vi "测试状态判断.vi"(10 "配置信息":T11, 11 "Display State In":T1) -> (1 "Data In":T3 caption="数据", 2 "配置信息读取":T11, 3 "Display State Out":T1)   [LabVIEW 2016, in "定时设置.xctl"]
uses:
  <vilib>/ptbypt/NI_PtbyPt.lvlib
panel:
  # "分钟"
  # "次"
  # "分钟"
  # "次"
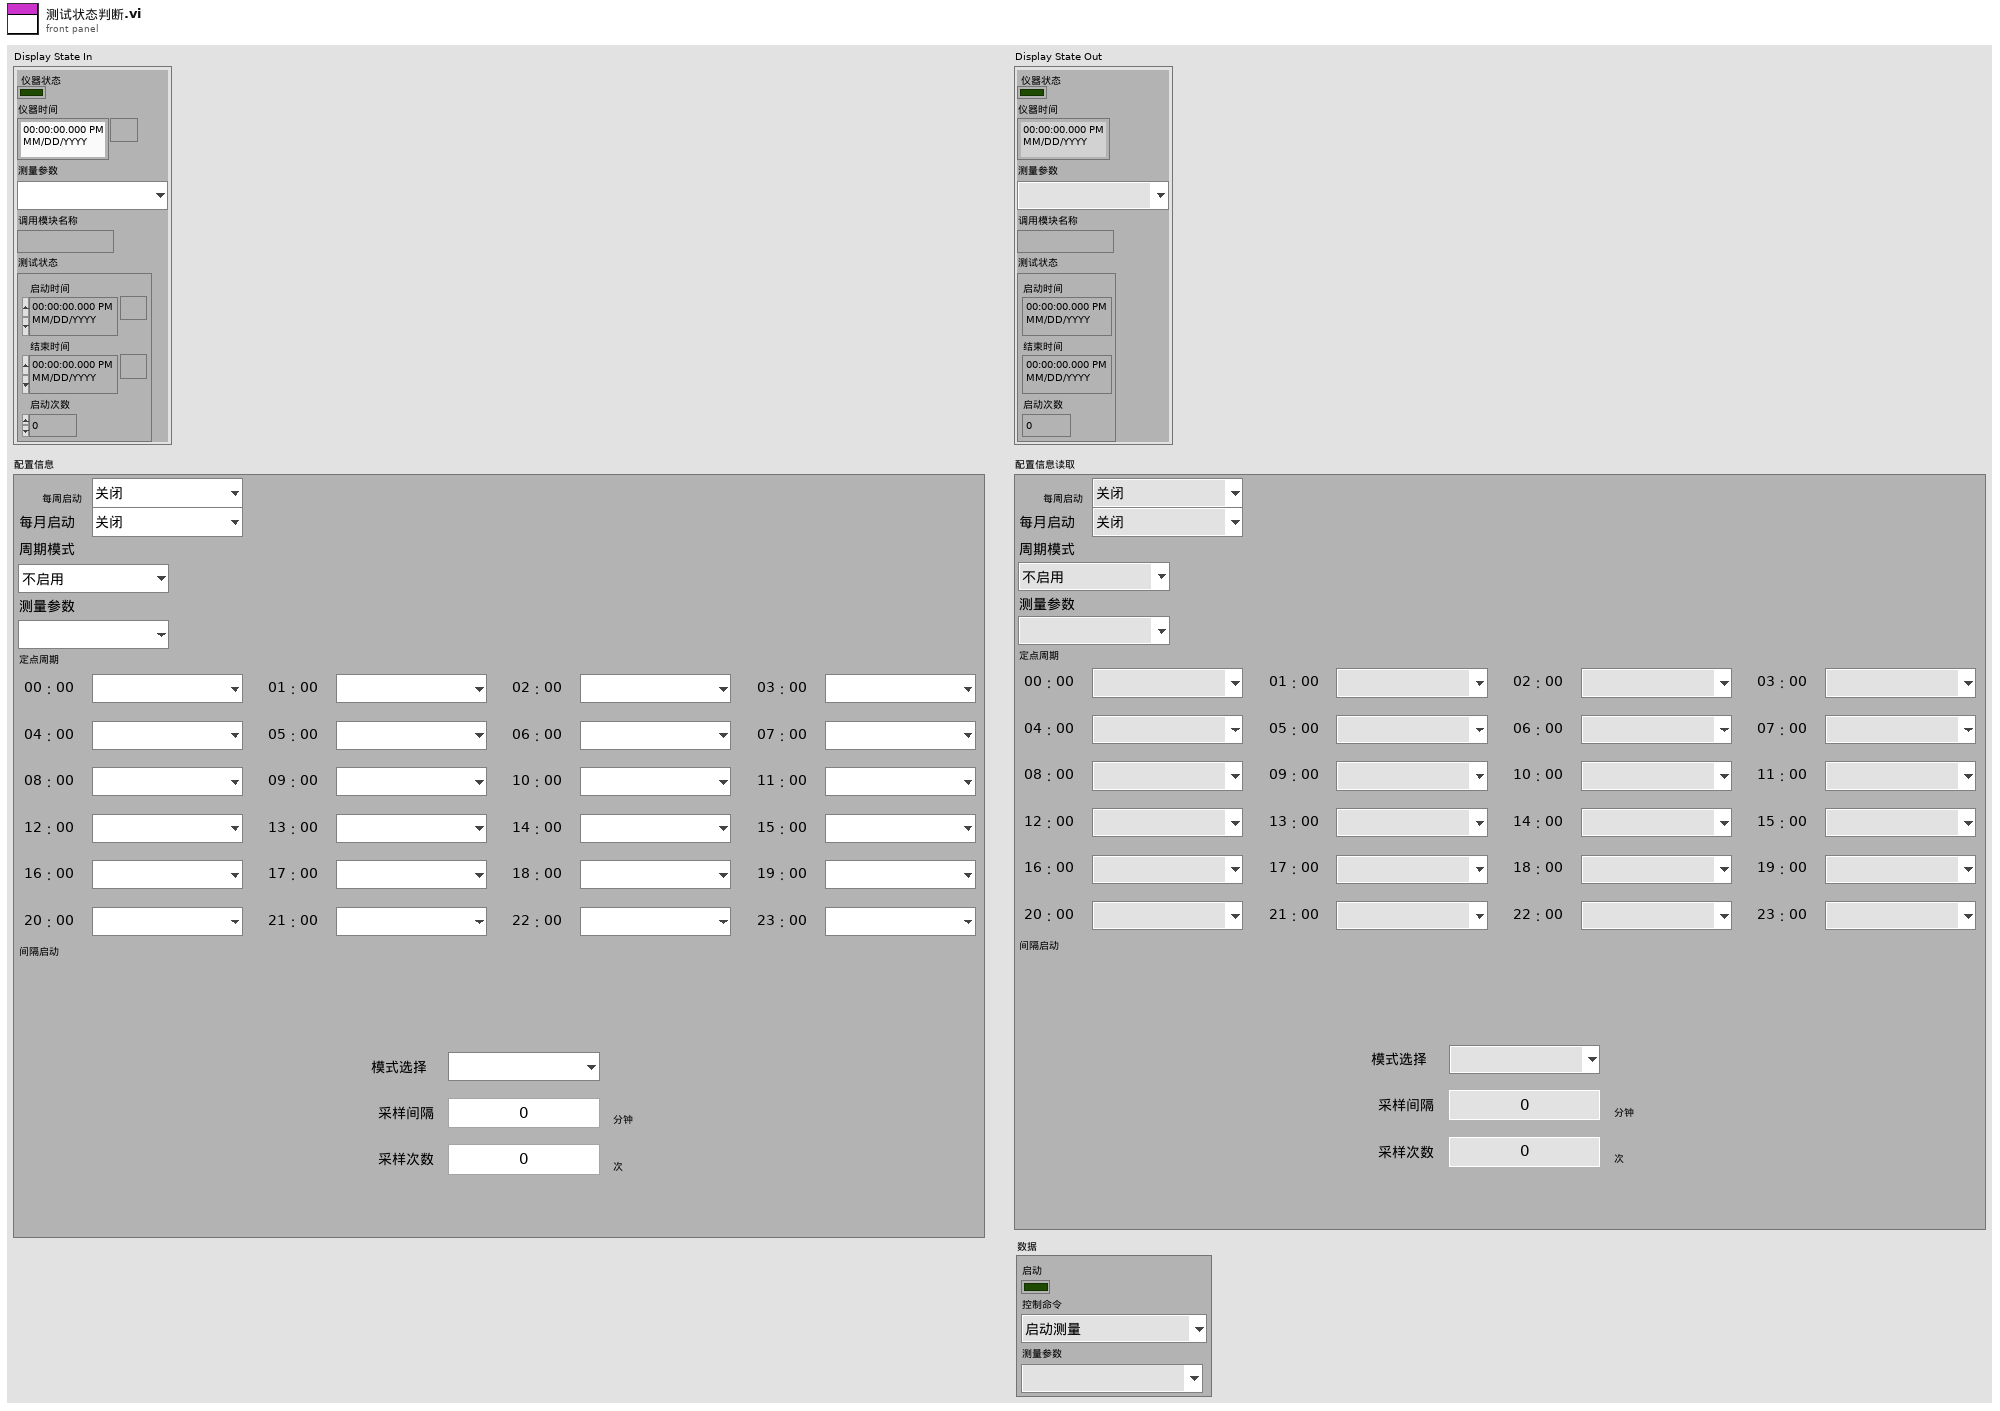
[diagram p1: front panel]
types:
  T1 = typedef "定时设置.xctl/状态 1.ctl" = cluster{"仪器状态":bool, "仪器时间":timestamp, "测量参数":T2, "调用模块名称":string, "测试状态":cluster{"启动时间":timestamp, "结束时间":timestamp, "启动次数":dbl}}
  T2 = typedef "定时设置.xctl/测量参数.ctl" = u16
  T3 = typedef "定时设置.xctl/数据 1.ctl" = cluster{"启动":bool, "控制命令":T4, "测量参数":T2}
  T4 = typedef "定时设置.xctl/国标控制命令.ctl" = enum16{"启动测量", "标样核查", "零点核查", "跨度核查", "空白测试", "平行样测试", "加标回收", "空白校准", "标样校准", "初始化（清洗）", "停止测试", "仪器重启", "校时", "模式设置", "测量间隔设置"}
  T5 = typedef "定时设置.xctl/每周启动.ctl" = enum16{"关闭", "周日", "周一", "周二", "周三", "周四", "周五", "周六"}
  T6 = typedef "定时设置.xctl/每月启动.ctl" = enum16{"关闭", "1号", "2号", "3号", "4号", "5号", "6号", "7号", "8号", "9号", "10号", "11号", "12号", "13号", "14号", "15号", "16号", "17号", "18号", "19号", "20号", "21号", "22号", "23号", "24号", "25号", "26号", "27号", "28号", "29号", "30号", "31号"}
  T7 = typedef "定时设置.xctl/周期模式设置.ctl" = enum16{"不启用", "定点模式", "间隔模式"}
  T8 = typedef "定时设置.xctl/定点周期设置.ctl" = cluster{"启动命令":T9, "启动命令 2":T9, "启动命令 3":T9, "启动命令 4":T9, "启动命令 5":T9, "启动命令 6":T9, "启动命令 7":T9, "启动命令 8":T9, "启动命令 9":T9, "启动命令 10":T9, "启动命令 11":T9, "启动命令 12":T9, "启动命令 13":T9, "启动命令 14":T9, "启动命令 15":T9, "启动命令 16":T9, "启动命令 17":T9, "启动命令 18":T9, "启动命令 19":T9, "启动命令 20":T9, "启动命令 21":T9, "启动命令 22":T9, "启动命令 23":T9, "启动命令 24":T9}
  T9 = typedef "定时设置.xctl/启动命令选择.ctl" = enum16{"", "水样测试", "标样核查", "零点核查", "跨度核查", "空白测试", "平行样测试", "加标回收", "空白校准", "标样校准", "初始化(清洗)"}
  T10 = typedef "定时设置.xctl/间隔启动设置.ctl" = cluster{"启动命令":T9, "启动间隔":dbl, "启动次数":i32}
  T11 = cluster{"每周启动":T5, "每月启动":T6, "周期模式":T7, "测量参数":T2, "定点周期":T8, "间隔启动":T10}
  T12 = typedef "LVDateTimeRec.ctl" = cluster{"秒数的小数部分":dbl, "秒":i32, "分":i32, "时":i32, "日":i32, "月":i32, "年":i32, "天数（周）":i32, "天数（年）":i32, "DST":i32}
  T13 = cluster{"启动时间":timestamp, "结束时间":timestamp, "启动次数":dbl}
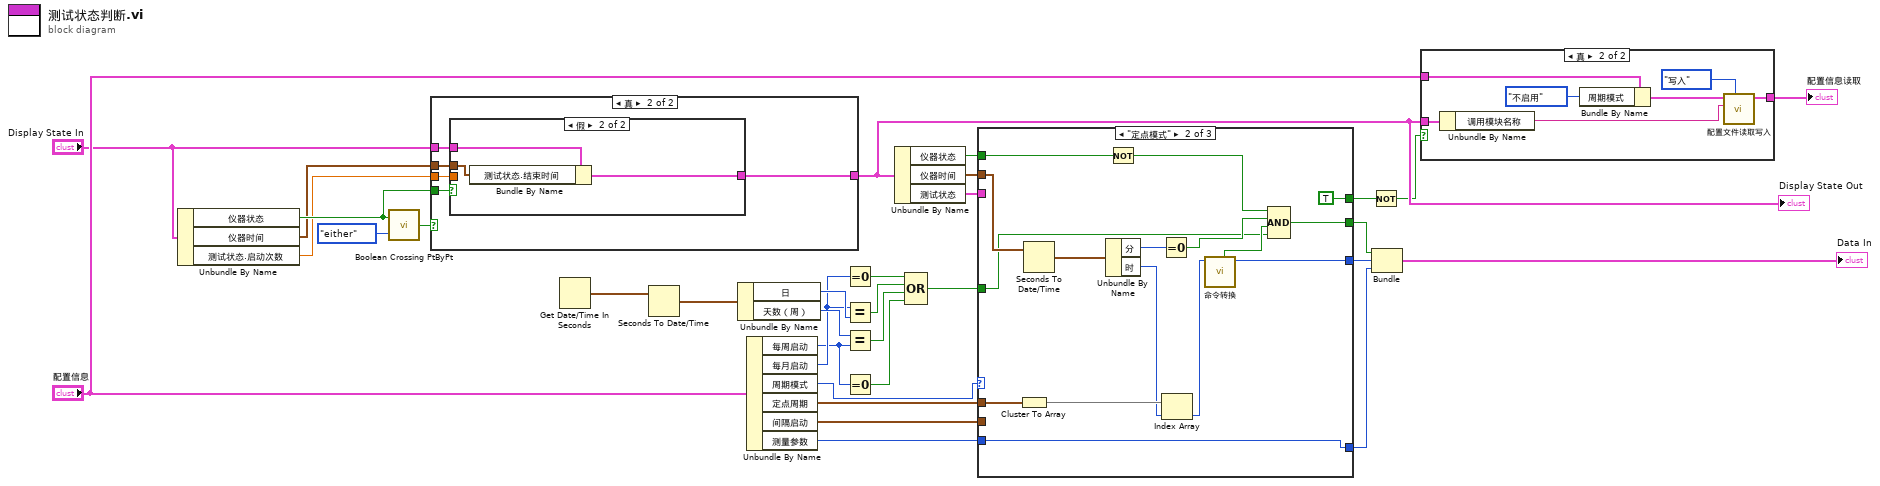
[diagram p0: block diagram]
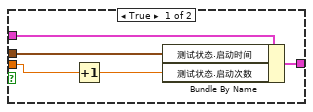
[diagram p4: hidden frame]
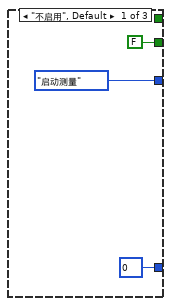
[diagram p5: hidden frame]
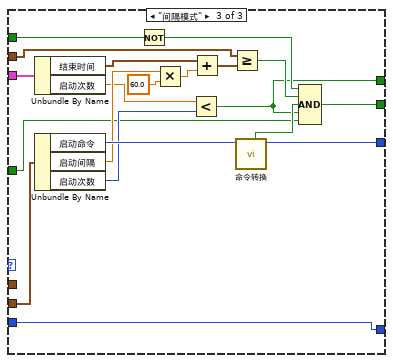
[diagram p6: hidden frame]
diagram:
  n1 = Unbundle By Name("Display State In") -> ("仪器状态"=w22:bool, "仪器时间"=w17:timestamp, "测试状态.启动次数"=w16:dbl)
  n2 = call <vilib>:"Boolean Crossing PtByPt.vi"("direction"=enum16{"either", "false-true", "true-false"}."either", "input"=w22) -> ("crossing"=w23:bool)  [unwired: 1 in]
  n3 = case shown="真" w23 {
    tunnel: "Display State In" -> [w34 w37]
    tunnel: [w34 w39] -> w13
    tunnel: w22 -> [_ w38]
    tunnel: w17 -> [_ w36]
    tunnel: w16 -> [_ w35]
    frame False {
    }
    frame True {
      n4 = case shown="假" w38 {
        tunnel: w37 -> [w42 w47]
        tunnel: w36 -> [w44 w46]
        tunnel: [w43 w45] -> w39
        tunnel: w35 -> [w40 _]
        frame True {
          n5 = Increment(x=w40) -> (x+1=w41:dbl)
          n6 = Bundle By Name(cluster=w42, "测试状态.启动时间"=w44, "测试状态.启动次数"=w41) -> (w43:T1)
        }
        frame False {
          n7 = Bundle By Name(cluster=w47, "测试状态.结束时间"=w46) -> (w45:T1)
        }
      }
    }
  }
  "Display State Out" <- w13
  n8 = Get Date/Time In Seconds() -> (seconds since 1Jan1904=w7:timestamp)
  n9 = Seconds To Date/Time(time stamp (now)=w7) -> (date time rec=w11:T12)  [unwired: 1 in]
  n10 = Unbundle By Name(w11) -> ("日"=w6:i32, "天数（周）"=w10:i32)
  n11 = Unbundle By Name("配置信息") -> ("每周启动"=w3:T5, "每月启动"=w5:T6, "周期模式"=w33:T7, "定点周期"=w31:T8, "间隔启动"=w30:T10, "测量参数"=w29:T2)
  n12 = Equal To 0?(x=w5) -> (x = 0?=w4:bool)
  n13 = Equal?(x=w5, y=w6) -> (x = y?=w9:bool)
  n14 = Equal?(x=w10, y=w3) -> (x = y?=w8:bool)
  n15 = Equal To 0?(x=w3) -> (x = 0?=w2:bool)
  n16 = Unbundle By Name(w13) -> ("仪器状态"=w18:bool, "仪器时间"=w19:timestamp, "测试状态"=w20:T13)
  n17 = Compound Arithmetic op=OR ("复合运算")(w4, w9, w8, w2) -> (w1:bool)
  n18 = case shown="\"定点模式\"" w33 {
    tunnel: w31 -> [_ w54 _]
    tunnel: w30 -> [_ _ w79]
    tunnel: w19 -> [_ w66 w72]
    tunnel: w18 -> [_ w63 w86]
    tunnel: w29 -> [_ w59 w82]
    tunnel: [国标控制命令."启动测量" ("控制命令") w57 w80] -> w27
    tunnel: [FALSE w60 w83] -> w28
    tunnel: [w48 w59 w82] -> w26
    tunnel: w20 -> [_ _ w78]
    tunnel: [_ TRUE w68] -> w14
    tunnel: w1 -> [_ w56 w67]
    frame "不启用", Default {
      w48 = T2 0 items=[""] ("测量参数")
    }
    frame "定点模式" {
      n19 = Cluster To Array(cluster=w54) -> (array=w53:T9[])
      n20 = Seconds To Date/Time(time stamp (now)=w66) -> (date time rec=w65:T12)  [unwired: 1 in]
      n21 = Unbundle By Name(w65) -> ("分"=w64:i32, "时"=w52:i32)
      n22 = Not(x=w63) -> (.not. x?=w62:bool)
      n23 = Equal To 0?(x=w64) -> (x = 0?=w61:bool)
      n24 = Index Array(array=w53, index=w52) -> (element=w51:T9)
      n25 = call "命令转换.vi"("启动命令"=w51) -> ("控制命令"=w57:T4, "布尔"=w58:bool)  [unwired: 9 in]
      n26 = Compound Arithmetic op=AND ("复合运算")(w62, w61, w58, w56) -> (w60:bool)
    }
    frame "间隔模式" {
      n27 = Unbundle By Name(w78) -> ("结束时间"=w77:timestamp, "启动次数"=w70:dbl)
      n28 = Unbundle By Name(w79) -> ("启动命令"=w84:T9, "启动间隔"=w76:dbl, "启动次数"=w69:i32)
      n29 = Not(x=w86) -> (.not. x?=w85:bool)
      n30 = Multiply(x=w76, y=60.0) -> (x*y=w74:dbl)
      n31 = Less?(x=w70, y=w69) -> (x < y?=w68:bool)
      n32 = Add(x=w77, y=w74) -> (x+y=w73:timestamp)
      n33 = Greater Or Equal?(x=w72, y=w73) -> (x >= y?=w71:bool)
      n34 = call "命令转换.vi"("启动命令"=w84) -> ("控制命令"=w80:T4, "布尔"=w81:bool)  [unwired: 9 in]
      n35 = Compound Arithmetic op=AND ("复合运算")(w85, w71, w81, w68, w67) -> (w83:bool)
    }
  }
  n36 = Not(x=w14) -> (.not. x?=w12:bool)
  n37 = Bundle(w28, "控制命令"=w27, "测量参数"=w26) -> (→"Data In":cluster{bool, "控制命令":T4, "测量参数":T2})  [unwired: 1 in]
  n38 = case shown="真" w12 {
    tunnel: "配置信息" -> [w87 w94]
    tunnel: [w87 w91] -> w15
    tunnel: w13 -> [_ w89]
    frame False {
    }
    frame True {
      n39 = Unbundle By Name(w89) -> ("调用模块名称"=w88:string)
      n40 = Bundle By Name(cluster=w94, "周期模式"=周期模式设置."不启用") -> (w92:T11)
      n41 = call "配置文件读取写入.vi"("配置模式"=enum16{"读取", "写入"}."写入", "配置文件名"=w88, "配置信息"=w92) -> ("配置信息读取"=w91:T11)  [unwired: 7 in, 1 out]
    }
  }
  "配置信息读取" <- w15
